vi "Get Color Index.vi"(5 "Bottom Color Ref":refnum<vi>, 7 "Top Color Ref":refnum<vi>, 8 "error in (no error)":errorcluster, 10 "Color Ref Array":refnum<vi>[](array[refnum]), 11 "Slider Ref Array":refnum<vi>[](array[refnum])) -> (0 "error out":errorcluster, 1 "Color Ramp Index":i32[](array[numeric]), 3 "Color Ramp Array":u32[](array[numeric]))   [LabVIEW 2017, in "3D Plot.lvclass"]
uses:
  <vilib>/Math Plots/3D Math Plots/3D Plot/3D Plot/3D Plot.lvclass
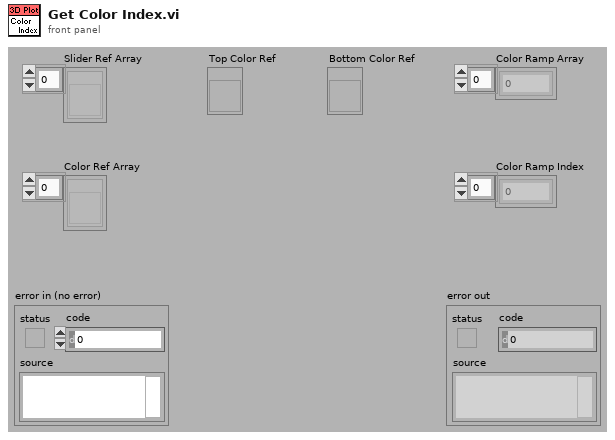
[diagram p1: front panel]
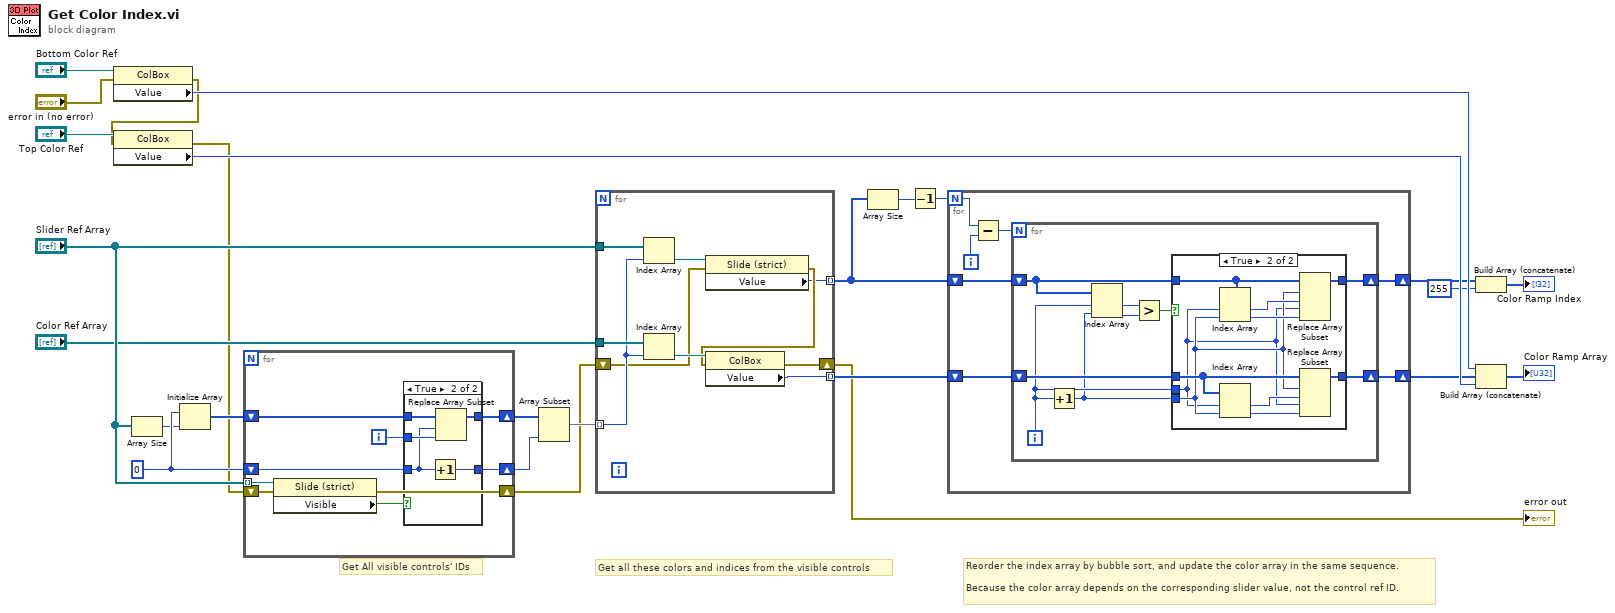
[diagram p0: block diagram]
diagram:
  w26 = 0
  # "Reorder the index array by bubble sort, and update the color array in the same sequence.\n\nBecause the color array depends on the corresponding slider value, not the control ref ID."
  # "Get all these colors and indices from the visible controls"
  # "Get All visible controls' IDs"
  n1 = property class="ColBox"(reference="Bottom Color Ref", error in="error in (no error)") -> (error out=w4:errorcluster, "Value"=w15:u32)  [unwired: 1 out]
  n2 = property class="ColBox"(reference="Top Color Ref", error in=w4) -> (error out=w3:errorcluster, "Value"=w14:u32)  [unwired: 1 out]
  n3 = Array Size(array="Slider Ref Array") -> (size(s)=w24:i32)
  n4 = Initialize Array(w26, w24) -> (w25:i32[])
  n5 = for {
    tunnel: "Slider Ref Array" -> [w34] mode=indexing
    shift-right: [w33] -> w22
    shift-left: w26 -> [w32]
    shift-right: [w30] -> w23
    shift-left: w25 -> [w31]
    shift-right: [w27] -> w2
    shift-left: w3 -> [w28]
    i -> [w29]
    n6 = property class="Slide (strict)"(reference=w34, error in=w28) -> (error out=w27:errorcluster, "Visible"=w35:bool)  [unwired: 1 out]
    n7 = case shown="True" w35 {
      tunnel: [w36 w42] -> w33
      tunnel: w32 -> [w36 w38]
      tunnel: w31 -> [w37 w41]
      tunnel: [w37 w40] -> w30
      tunnel: w29 -> [_ w39]
      frame False {
      }
      frame True {
        n8 = Increment(x=w38) -> (x+1=w42:i32)
        n9 = Replace Array Subset(array=w41, new element=w39, index=w38) -> (w40:i32[])
      }
    }
  }
  n10 = Array Subset(array=w23, length=w22) -> (w21:i32[])  [unwired: 1 in]
  n11 = for {
    tunnel: w21 -> [w47] mode=indexing
    tunnel: "Slider Ref Array" -> [w52]
    tunnel: "Color Ref Array" -> [w50]
    tunnel: [w48] -> w18 mode=indexing
    tunnel: [w43] -> w9 mode=indexing
    shift-right: [w44] -> w1
    shift-left: w2 -> [w46]
    n12 = Index Array(array=w52, index=w47) -> (element=w51:refnum<vi>)
    n13 = Index Array(array=w50, index=w47) -> (element=w49:refnum<vi>)
    n14 = property class="Slide (strict)"(reference=w51, error in=w46) -> (error out=w45:errorcluster, "Value"=w43:i32)  [unwired: 1 out]
    n15 = property class="ColBox"(reference=w49, error in=w45) -> (error out=w44:errorcluster, "Value"=w48:u32)  [unwired: 1 out]
  }
  "error out" <- w1
  n16 = Array Size(array=w9) -> (size(s)=w10:i32)
  n17 = Decrement(x=w10) -> (x-1=w6:i32)
  n18 = for {
    N: w6 -> [w55]
    shift-right: [w57] -> w8
    shift-left: w9 -> [w59]
    shift-right: [w56] -> w7
    shift-left: w18 -> [w58]
    i -> [w54]
    n19 = Subtract(x=w55, y=w54) -> (x-y=w53:i32)
    n20 = for {
      N: w53 -> [_]
      shift-right: [w64] -> w57
      shift-left: w59 -> [w66]
      shift-right: [w63] -> w56
      shift-left: w58 -> [w62]
      i -> [w61]
      n21 = Increment(x=w61) -> (x+1=w60:i32)
      n22 = Index Array(array=w66, index #1=w61, index #2=w60) -> (element #1=w68:i32, element #2=w67:i32)
      n23 = Greater?(x=w68, y=w67) -> (0:w65:bool)
      n24 = case shown="True" w65 {
        tunnel: w66 -> [w70 w80]
        tunnel: [w70 w79] -> w64
        tunnel: [w69 w77] -> w63
        tunnel: w62 -> [w69 w78]
        tunnel: w61 -> [_ w71]
        tunnel: w60 -> [_ w72]
        frame False {
        }
        frame True {
          n25 = Index Array(array=w80, index #1=w71, index #2=w72) -> (element #1=w76:i32, element #2=w75:i32)
          n26 = Index Array(array=w78, index #1=w71, index #2=w72) -> (element #1=w73:u32, element #2=w74:u32)
          n27 = Replace Array Subset(array=w80, new element #1=w76, index #1=w72, new element #2=w75, index #2=w71) -> (w79:i32[])
          n28 = Replace Array Subset(array=w78, new element #1=w73, index #1=w72, new element #2=w74, index #2=w71) -> (w77:u32[])
        }
      }
    }
  }
  n29 = Build Array (concatenate)(w8, 255) -> (→"Color Ramp Index":i32[])
  n30 = Build Array (concatenate)(w15, w7, w14) -> (→"Color Ramp Array":u32[])
